vi "XML Script - Function.vi"   [LabVIEW 2020]
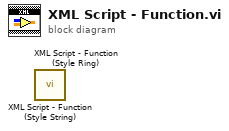
[diagram p0: block diagram]
diagram:
  n1 = call <vilib>:"XML Script - Function (Style String).vi"() -> ()  [unwired: 10 in, 2 out]
  n2 = call <vilib>:"XML Script - Function (Style Ring).vi"() -> ()  [unwired: 10 in, 2 out]
